vi "fpga_DAC_sine.vi"() -> ()   [LabVIEW 2018]
uses:
  <vilib>/rvi/FXPMathLib/FxpSinAndCos/subVIs/nifxpmath_SinAndCos_SimConfig.ctl
  <vilib>/rvi/Emulation/niFpgaGetClockAttributes.vi
  <vilib>/rvi/Emulation/niFpgaSctlEmulationGetInTimedLoop.vi
  <vilib>/rvi/Emulation/niFpgaEmulationReportErrorSimple.vi
  <vilib>/rvi/eio/common/nirviEmuTemplateMethod_errors.vi
  <vilib>/rvi/FXPMathLib/FxpSinAndCos/simVIs/DllFxpSinAndCosTemp_sub.vi
  <vilib>/rvi/Emulation/niFpgaCriticalErrorInLSC.vi
  <vilib>/eio/EIONode/EIONode.xnode
  <vilib>/rvi/FXPMathLib/FxpSinAndCos/XNode/nifxpmath_SinAndCos.xnode
panel:
  out "0":fxp<+,52,36> format="%.27g"
  out "2":fxp<+/-,16,2> format="%.15g"
  out "1":fxp<+/-,33,14> format="%.24g"
  in  "freq (Hz)":fxp<+,20,16>
  in  "offset (V)":i16
  in  "amplitude (V)":i16=2018
  in  "datapoints/cycle":u16=2000
  out "binary":bool[](array[boolean])
  # "Probes"
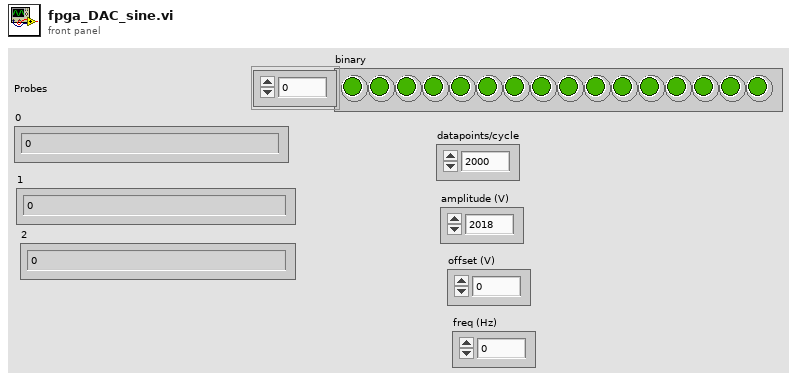
[diagram p1: front panel]
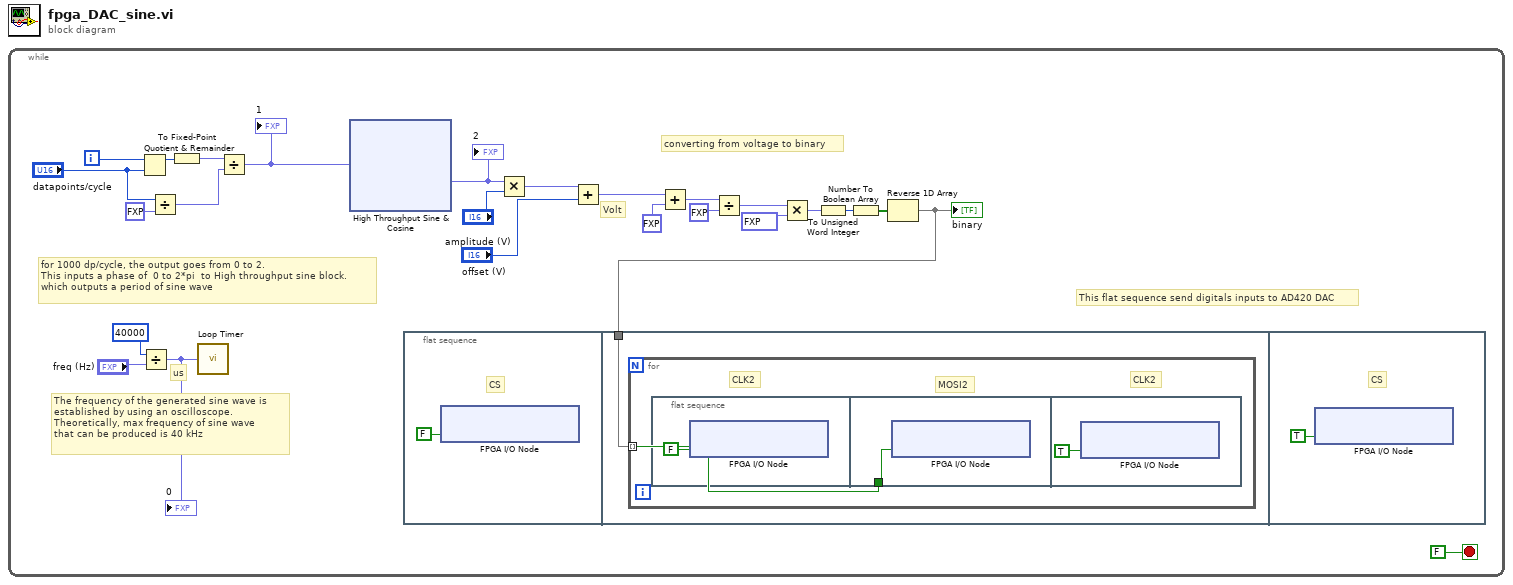
[diagram p0: block diagram]
diagram:
  n1 = while {
    i -> [w14]
    stop <- FALSE stop-if-true
    # "converting from voltage to binary"
    # "This flat sequence send digitals inputs to AD420 DAC"
    # "us"
    # "The frequency of the generated sine wave is \nestablished by using an oscilloscope. \nTheoretically, max frequency of sine wave \nthat can be produced is 40 kHz"
    # "Volt"
    # "for 1000 dp/cycle, the output goes from 0 to 2.\nThis inputs a phase of  0 to 2*pi  to High throughput sine block.\nwhich outputs a period of sine wave"
    n2 = Quotient & Remainder(x=w14, y="datapoints/cycle") -> (x-y*floor(x/y)=w13:i32)  [unwired: 1 out]
    n3 = Divide(x=u32 40000, y="freq (Hz)") -> (x/y=w2:fxp<+,52,36>)
    "0" <- w2
    n4 = Divide(x="datapoints/cycle", y=fxp<+,1,2> 2.0) -> (x/y=w5:fxp<+,17,15>)
    n5 = To Fixed-Point(number=w13) -> (fixed-point=w7:fxp<+/-,16,12>)  [unwired: 1 in]
    n6 = call "Loop Timer"("Count(Ticks)"=w2) -> ()  [unwired: 1 out]
    n7 = Divide(x=w7, y=w5) -> (x/y=w12:fxp<+/-,33,14>)
    "1" <- w12
    n8 = xnode "High Throughput Sine & Cosine"("x (pi)"=w12) -> ("sin(x)"=w11:fxp<+/-,16,2>)  [unwired: 1 out]
    "2" <- w11
    n9 = flat-sequence {
      tunnel: w18 -> [w57]
      frame #0 {
        # "CS"
        n10 = xnode "FPGA I/O Node"("ConnectorA/DIO4"=FALSE) -> ()  [unwired: 1 in, 1 out]
      }
      frame #1 {
        n11 = for {
          tunnel: w57 -> [w58] mode=indexing
          # "CLK2"
          # "CLK2"
          # "MOSI2"
          n12 = flat-sequence {
            tunnel: w58 -> [w60]
            frame #0 {
              n13 = xnode "FPGA I/O Node"("ConnectorA/DIO5"=FALSE) -> ()  [unwired: 1 in, 1 out]
            }
            frame #1 {
              n14 = xnode "FPGA I/O Node"("ConnectorA/DIO6"=w60) -> ()  [unwired: 1 in, 1 out]
            }
            frame #2 {
              n15 = xnode "FPGA I/O Node"("ConnectorA/DIO5"=TRUE) -> ()  [unwired: 1 in, 1 out]
            }
          }
        }
      }
      frame #2 {
        # "CS"
        n16 = xnode "FPGA I/O Node"("ConnectorA/DIO4"=TRUE) -> ()  [unwired: 1 in, 1 out]
      }
    }
    n17 = Multiply(x=w11, y="amplitude (V)") -> (x*y=w16:fxp<+/-,32,18>)
    n18 = Add(x=w16, y="offset (V)") -> (x+y=w10:fxp<+/-,32,18>)
    n19 = Add(x=w10, y=fxp<+,3,4> 10.0) -> (x+y=w23:fxp<+/-,32,18>)
    n20 = Divide(x=w23, y=fxp<+,3,5> 20.0) -> (x/y=w9:fxp<+/-,33,14>)
    n21 = Multiply(x=w9, y=fxp<+,16,16> 65535.0) -> (x*y=w8:fxp<+/-,49,30>)
    n22 = To Unsigned Word Integer(number=w8) -> (unsigned 16bit integer=w21:u16)
    n23 = Number To Boolean Array(number=w21) -> (Boolean array=w20:bool[])
    n24 = Reverse 1D Array(array=w20) -> (reversed array=w18:bool[])
    "binary" <- w18
  }
